vi "Cloud Data Processor v3.vi"(11 "file path (dialog if empty)":path) -> (0 "Humidity":i32[](array[numeric]), 1 "Light":dbl[](array[numeric]), 3 "Temperature":i32[](array[numeric]))   [LabVIEW 2014]
uses:
  <vilib>/Utility/file.llb/Read From Spreadsheet File (string).vi
panel:
  in  "?":enum32{"Temperature", "Humidity", "Light"}(tab)
  out "Min < 60°F?":bool
  out "Max > 80°F?":bool
  out "Maximum Temperature (°F)":dbl
  out "Temperature Readings":i32[](graph)
  out "Running Average Temperature":dbl(graph)
  out "Minimum Temperature (°F)":dbl
  out "Average Temperature (°F)":dbl
  out "Humidity Readings":i32[](graph)
  out "Running Average Humidity":dbl(graph)
  out "Average Humidity (%)":dbl
  out "Maximum Humidity (%)":dbl
  out "Minimum Humidity (%)":dbl
  out "Max > 90%":bool
  out "Min < 40%":bool
  out "Light Readings":dbl[](graph)
  out "Maximum Light (V)":dbl
  out "Minimum Light (V)":dbl
  out "Max > 4.0V":bool
  out "Min < 0.1V":bool
  out "Average Light (V)":dbl
  out "Running Average Light":dbl(graph)
  out "scrubbed humidity":string[](array[string])
  out "scrubbed light":string[](array[string])
  out "scrubbed temp":string[](array[string])
  out "Humidity":string[](array[string])
  out "Temperature":string[](array[string])
  out "Light":string[](array[string])
  out "Data":string[](array[string])
  out "labels":string[](array[string])
  out "all rows":string[][](array[string])
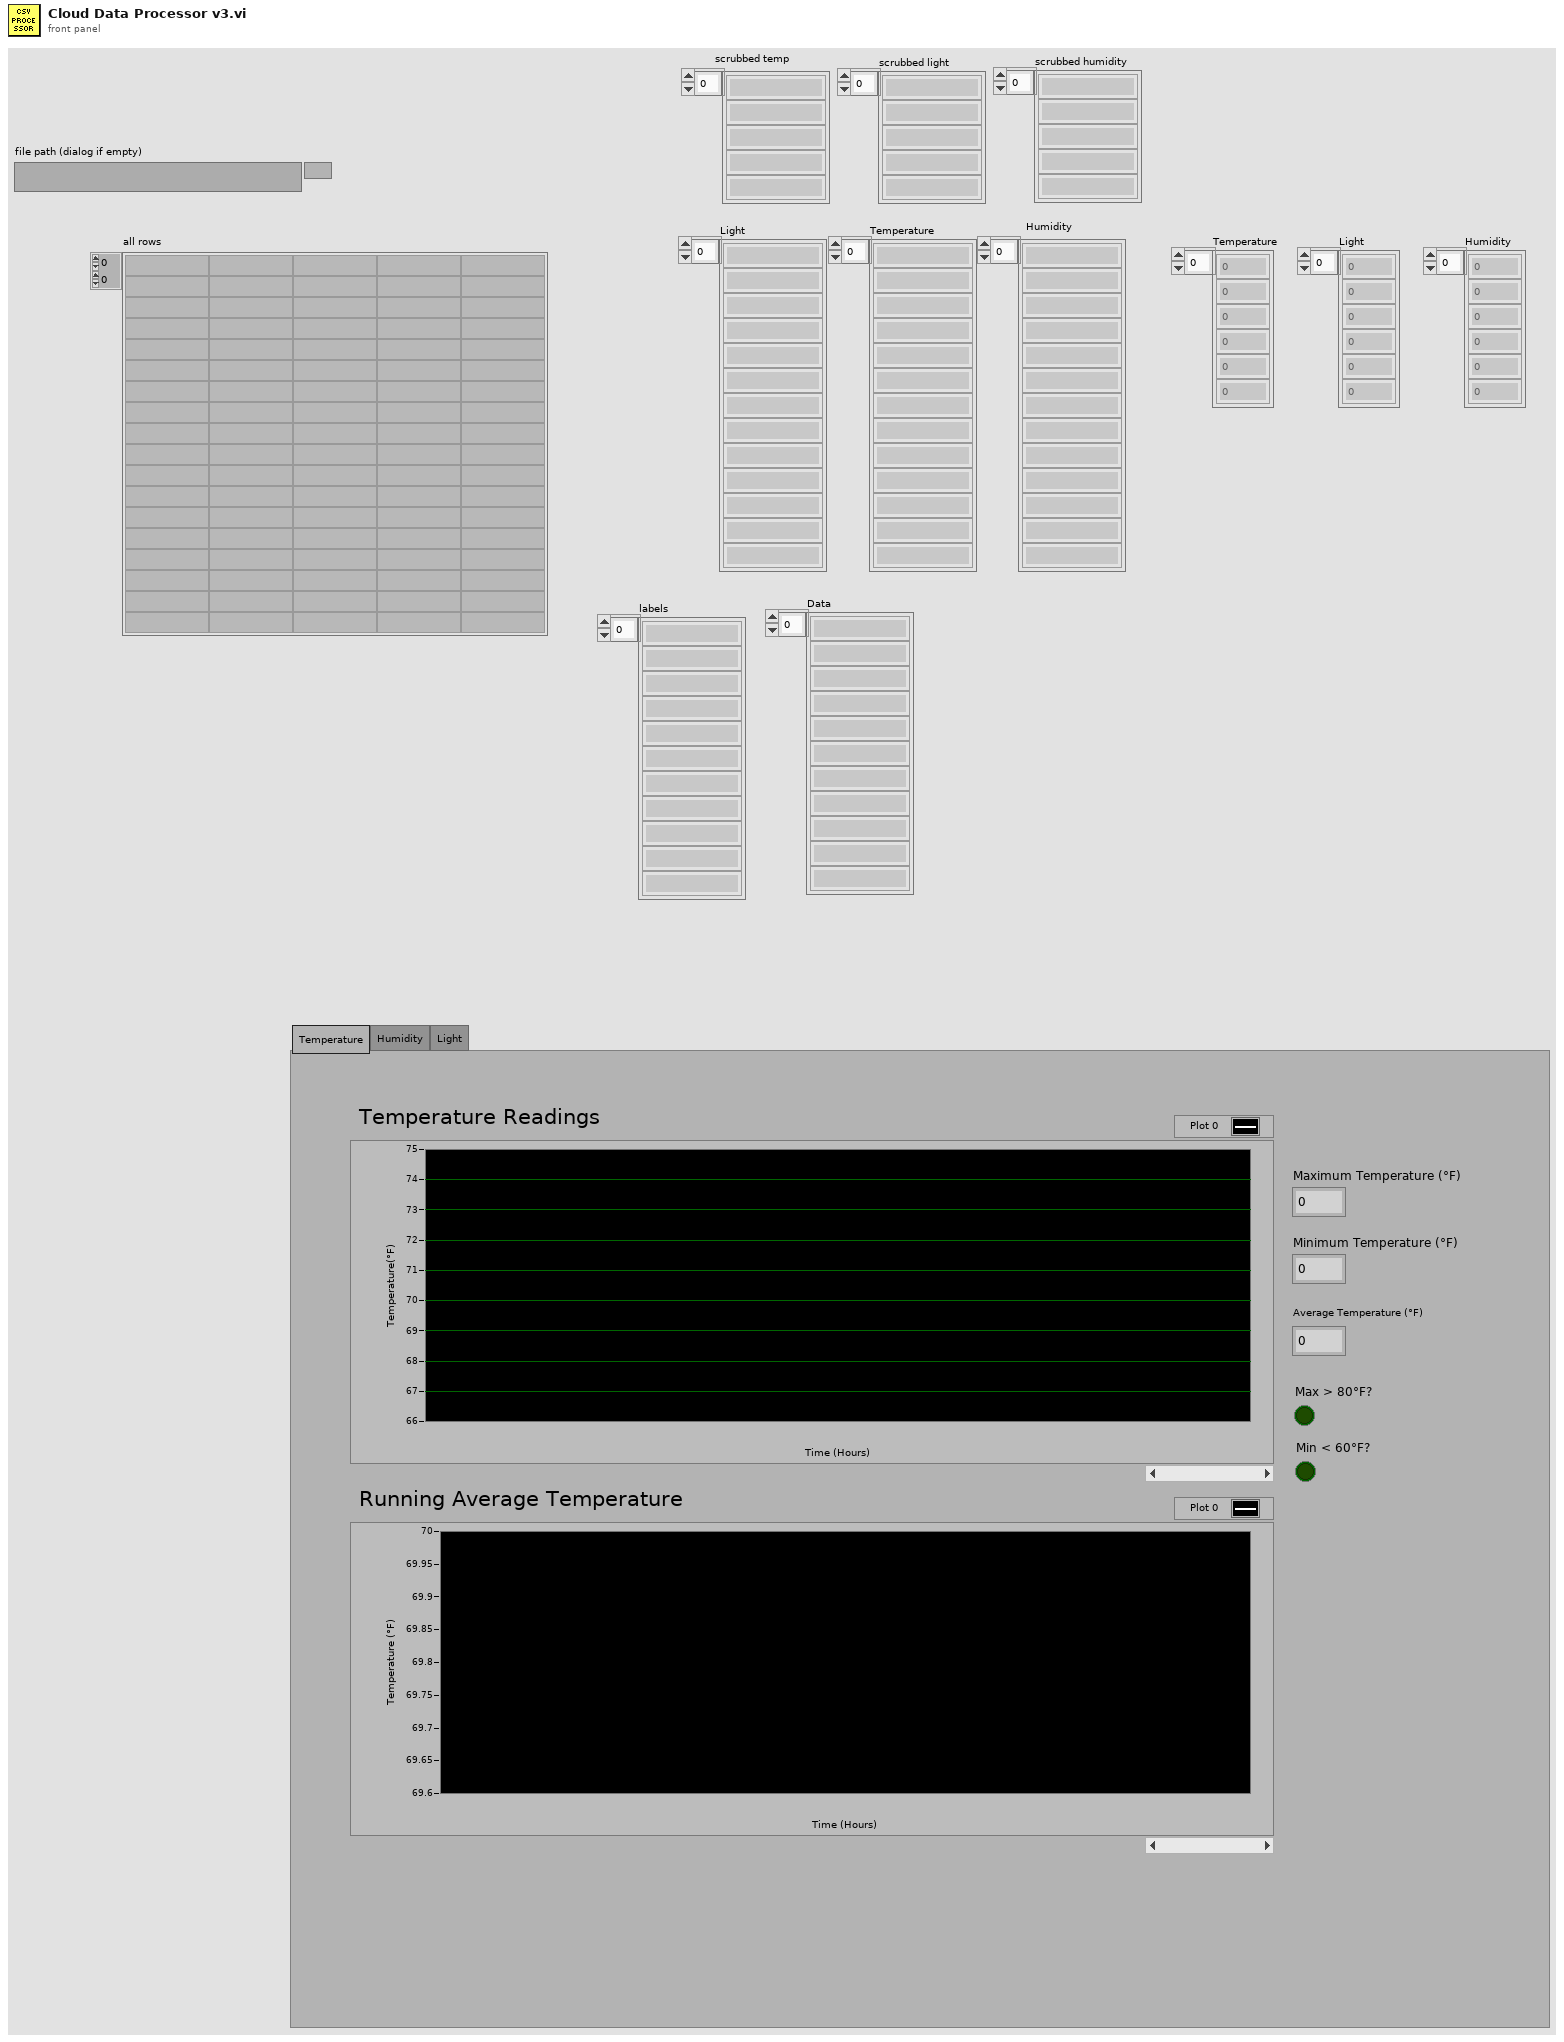
[diagram p1: front panel]
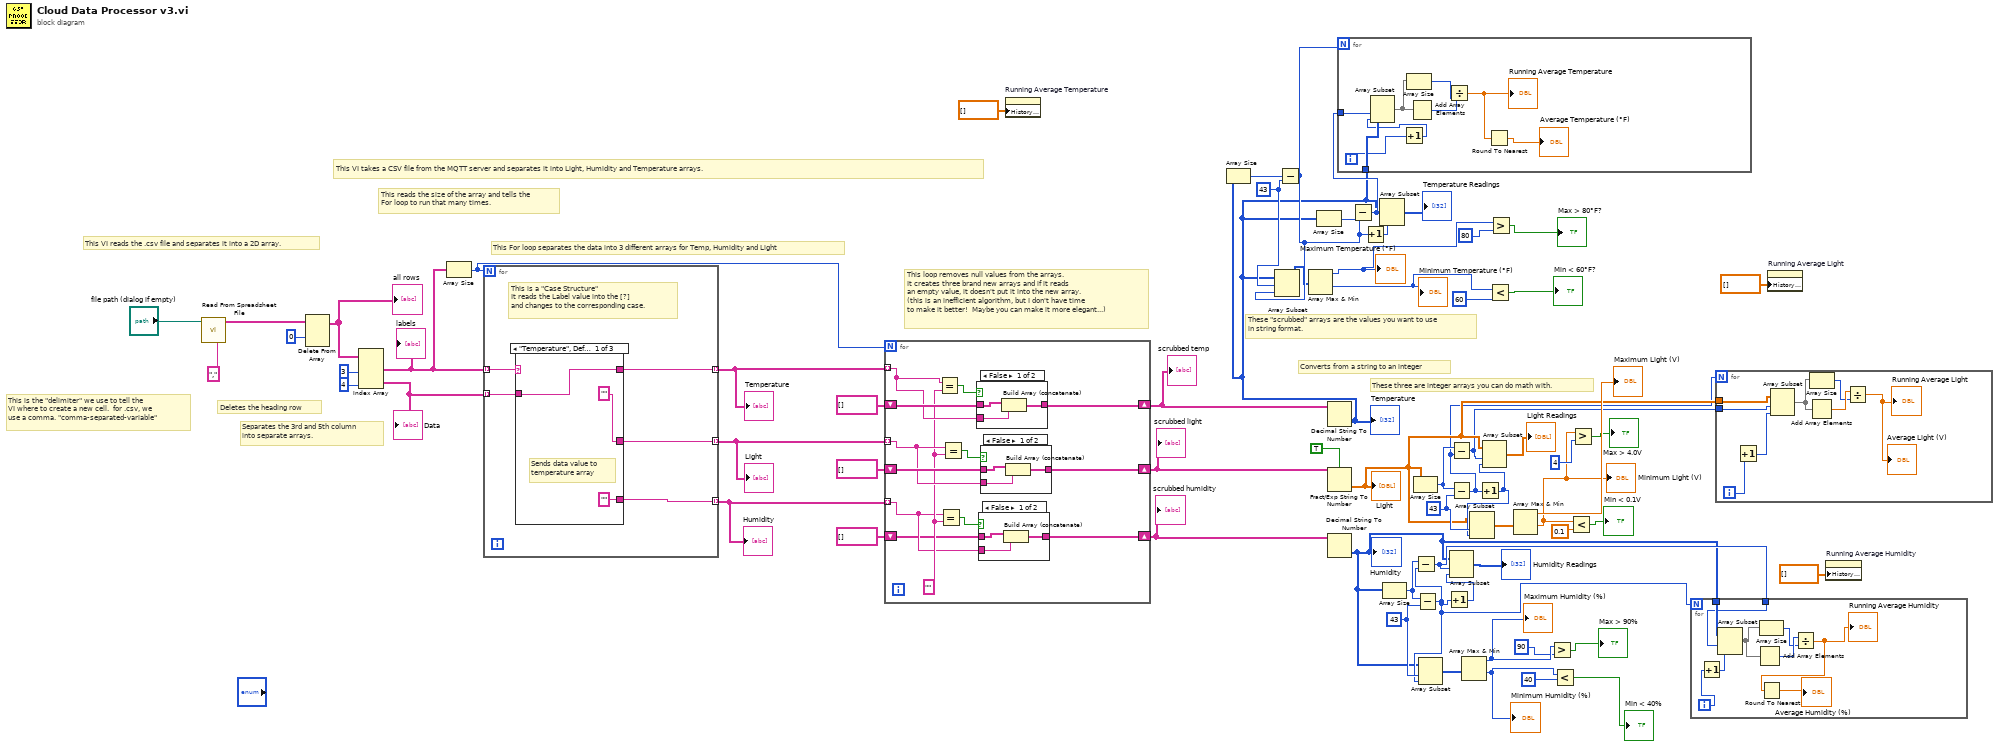
[diagram p0: block diagram]
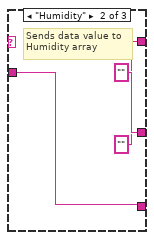
[diagram p5: hidden frame]
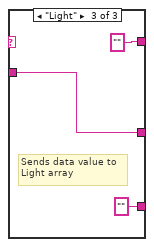
[diagram p6: hidden frame]
diagram:
  w13 = 43
  w30 = 43
  w39 = 43
  # "These three are integer arrays you can do math with."
  # "This VI takes a CSV file from the MQTT server and separates it into Light, Humidity and Temperature arrays."
  # "This is the \"delimiter\" we use to tell the\nVI where to create a new cell.  for .csv, we\nuse a comma. \"comma-separated-variable\""
  # "This VI reads the .csv file and separates it into a 2D array."
  # "This reads the size of the array and tells the\nFor loop to run that many times."
  # "Separates the 3rd and 5th column\ninto separate arrays."
  # "This For loop separates the data into 3 different arrays for Temp, Humidity and Light"
  # "Converts from a string to an integer"
  # "These \"scrubbed\" arrays are the values you want to use\nin string format."
  # "This loop removes null values from the arrays.\nIt creates three brand new arrays and if it reads\nan empty value, it doesn't put it into the new array.\n(this is an inefficient algorithm, but I don't have time\nto make it better!  Maybe you can make it more elegant...)"
  # "Deletes the heading row"
  n1 = call-poly <vilib>:"Read From Spreadsheet File.vi"("delimiter (\\t)"="," ("delimiter (\\t)"), "file path (dialog if empty)"="file path (dialog if empty)") -> ("all rows"=w62:string[][])  [unwired: 5 in, 4 out]
  n2 = Delete From Array(array=w62, index (row)=0) -> (array with subset deleted=w48:string[][])  [unwired: 2 in, 1 out]
  "all rows" <- w48
  n3 = Index Array(array=w48, index (col) #1=3 ("disabled index (col)"), index (col) #2=4 ("index (col)")) -> (element #1=w60:string[], element #2=w59:string[])  [unwired: 2 in]
  "labels" <- w60
  "Data" <- w59
  n4 = Array Size(array=w60) -> (size(s)=w47:i32)
  n5 = for {
    N: w47 -> [_]
    tunnel: w60 -> [w71] mode=indexing
    tunnel: w59 -> [w70] mode=indexing
    tunnel: [w69] -> w51 mode=indexing
    tunnel: [w68] -> w52 mode=indexing
    tunnel: [w67] -> w50 mode=indexing
    # "This is a \"Case Structure\"\nIt reads the Label value into the [?]\nand changes to the corresponding case."
    n6 = case shown="\"Temperature\", Default" w71 {
      tunnel: w70 -> [w74 w77 w80]
      tunnel: ["" ("String") "" ("String") w80] -> w69
      tunnel: [w74 "" ("String") "" ("String")] -> w68
      tunnel: ["" ("String") w77 "" ("String")] -> w67
      frame "Temperature", Default {
        # "Sends data value to \ntemperature array"
      }
      frame "Humidity" {
        # "Sends data value to \nHumidity array"
      }
      frame "Light" {
        # "Sends data value to \nLight array"
      }
    }
  }
  "Light" <- w51
  "Temperature" <- w52
  "Humidity" <- w50
  n7 = for {
    N: w47 -> [_]
    tunnel: w52 -> [w89] mode=indexing
    tunnel: w51 -> [w86] mode=indexing
    tunnel: w50 -> [w83] mode=indexing
    shift-right: [w92] -> w58
    shift-left: string[] [] -> [w91]
    shift-right: [w88] -> w57
    shift-left: string[] [] -> [w87]
    shift-right: [w82] -> w56
    shift-left: string[] [] -> [w81]
    w84 = "" ("String")
    n8 = Equal?(x=w89, y=w84) -> (x = y?=w93:bool)
    n9 = Equal?(x=w83, y=w84) -> (x = y?=w85:bool)
    n10 = Equal?(x=w86, y=w84) -> (x = y?=w90:bool)
    n11 = case shown="False" w93 {
      tunnel: w89 -> [w104 _]
      tunnel: [w103 w105] -> w92
      tunnel: w91 -> [w102 w105]
      frame False {
        n12 = Build Array (concatenate)(w102, w104) -> (w103:string[])
      }
      frame True {
      }
    }
    n13 = case shown="False" w85 {
      tunnel: w83 -> [w96 _]
      tunnel: [w95 w97] -> w82
      tunnel: w81 -> [w94 w97]
      frame False {
        n14 = Build Array (concatenate)(w94, w96) -> (w95:string[])
      }
      frame True {
      }
    }
    n15 = case shown="False" w90 {
      tunnel: w86 -> [w100 _]
      tunnel: [w99 w101] -> w88
      tunnel: w87 -> [w98 w101]
      frame False {
        n16 = Build Array (concatenate)(w98, w100) -> (w99:string[])
      }
      frame True {
      }
    }
  }
  "scrubbed temp" <- w58
  "scrubbed light" <- w57
  "scrubbed humidity" <- w56
  n17 = property on="Running Average Temperature" class="WFChart (strict)"("History Data"=dbl[] []) -> ()  [unwired: 2 in, 2 out]
  n18 = Decimal String To Number(string=w58) -> (number=w38:i32[])  [unwired: 2 in, 1 out]
  "Temperature" <- w38
  n19 = Array Size(array=w38) -> (size(s)=w41:i32)
  n20 = Subtract(x=w41, y=w39) -> (x-y=w40:i32)
  n21 = Array Subset(array=w38, index=w39, length=w40) -> (w37:i32[])
  n22 = Array Max & Min(array=w37) -> (max value=w33:i32, min value=w36:i32)  [unwired: 2 out]
  "Maximum Temperature (°F)" <- w33
  "Minimum Temperature (°F)" <- w36
  n23 = Array Size(array=w38) -> (size(s)=w44:i32)
  n24 = Fract/Exp String To Number(use system decimal point (T)=TRUE, string=w57) -> (number=w4:dbl[])  [unwired: 2 in, 1 out]
  "Light" <- w4
  n25 = Decimal String To Number(string=w56) -> (number=w17:i32[])  [unwired: 2 in, 1 out]
  "Humidity" <- w17
  n26 = Subtract(x=w44, y=w40) -> (x-y=w43:i32)
  n27 = for {
    N: w40 -> [_]
    tunnel: w38 -> [w114]
    tunnel: w43 -> [w113]
    i -> [w108]
    n28 = Increment(x=w108) -> (x+1=w109:i32)
    n29 = Array Subset(array=w114, index=w113, length=w109) -> (w112:i32[])
    n30 = Array Size(array=w112) -> (size(s)=w110:i32)
    n31 = Add Array Elements(numeric array=w112) -> (sum=w111:i32)
    n32 = Divide(x=w111, y=w110) -> (x/y=w107:dbl)
    "Running Average Temperature" <- w107
    n33 = Round To Nearest(number=w107) -> (nearest integer value=→"Average Temperature (°F)":dbl)
  }
  n34 = Increment(x=w40) -> (x+1=w46:i32)
  n35 = Array Subset(array=w38, index=w43, length=w46) -> (→"Temperature Readings":i32[])
  n36 = Array Size(array=w17) -> (size(s)=w22:i32)
  n37 = Array Size(array=w4) -> (size(s)=w15:i32)
  n38 = Subtract(x=w22, y=w30) -> (x-y=w19:i32)
  n39 = Subtract(x=w22, y=w19) -> (x-y=w18:i32)
  n40 = Array Subset(array=w17, index=w30, length=w19) -> (w29:i32[])
  n41 = Increment(x=w19) -> (x+1=w21:i32)
  n42 = Subtract(x=w15, y=w13) -> (x-y=w2:i32)
  n43 = Subtract(x=w15, y=w2) -> (x-y=w3:i32)
  n44 = Array Subset(array=w17, index=w18, length=w21) -> (→"Humidity Readings":i32[])
  n45 = Array Max & Min(array=w29) -> (max value=w28:i32, min value=w25:i32)  [unwired: 2 out]
  "Maximum Humidity (%)" <- w28
  "Minimum Humidity (%)" <- w25
  n46 = Increment(x=w2) -> (x+1=w12:i32)
  n47 = Array Subset(array=w4, index=w13, length=w12) -> (w11:dbl[])
  n48 = Array Subset(array=w4, index=w3, length=w12) -> (→"Light Readings":dbl[])
  n49 = Less?(x=w36, y=60) -> (x < y?=→"Min < 60°F?":bool)
  n50 = Greater?(x=w33, y=80) -> (0:→"Max > 80°F?":bool)
  n51 = Array Max & Min(array=w11) -> (max value=→"Maximum Light (V)":dbl, min value=w5:dbl)  [unwired: 2 out]
  "Minimum Light (V)" <- w5
  n52 = Greater?(x=w28, y=90) -> (0:→"Max > 90%":bool)
  n53 = Less?(x=w25, y=40) -> (x < y?=→"Min < 40%":bool)
  n54 = Less?(x=w5, y=0.1) -> (x < y?=→"Min < 0.1V":bool)
  n55 = Greater?(x=w5, y=4) -> (0:→"Max > 4.0V":bool)
  n56 = for {
    N: w19 -> [_]
    tunnel: w18 -> [w122]
    tunnel: w17 -> [w123]
    i -> [w121]
    n57 = Increment(x=w121) -> (x+1=w120:i32)
    n58 = Array Subset(array=w123, index=w122, length=w120) -> (w119:i32[])
    n59 = Add Array Elements(numeric array=w119) -> (sum=w116:i32)
    n60 = Array Size(array=w119) -> (size(s)=w115:i32)
    n61 = Divide(x=w116, y=w115) -> (x/y=w118:dbl)
    "Running Average Humidity" <- w118
    n62 = Round To Nearest(number=w118) -> (nearest integer value=→"Average Humidity (%)":dbl)
  }
  n63 = for {
    N: w2 -> [_]
    tunnel: w4 -> [w131]
    tunnel: w3 -> [w130]
    i -> [w129]
    n64 = Increment(x=w129) -> (x+1=w128:i32)
    n65 = Array Subset(array=w131, index=w130, length=w128) -> (w127:dbl[])
    n66 = Add Array Elements(numeric array=w127) -> (sum=w125:dbl)
    n67 = Array Size(array=w127) -> (size(s)=w124:i32)
    n68 = Divide(x=w125, y=w124) -> (x/y=→"Average Light (V)" →"Running Average Light":dbl)
  }
  n69 = property on="Running Average Light" class="WFChart (strict)"("History Data"=dbl[] []) -> ()  [unwired: 2 in, 2 out]
  n70 = property on="Running Average Humidity" class="WFChart (strict)"("History Data"=dbl[] []) -> ()  [unwired: 2 in, 2 out]
